vi "SwitchesMirrors.vi"(0 "Function":T5, 5 "Relay VISA Session":refnum<visa-resource-name>="COM1", 7 "Set Switch":T1, 9 "Delays (ms)":cluster{"Laser":u32, "Video":u32}={"Laser"=500, "Video"=1500}, 11 "Error In":errorcluster, 13 "Refnums":T4, 14 "Notifiers":T3) -> (8 "Get Switch":T1, 15 "Error Out":errorcluster)   [LabVIEW 2014]
uses:
  SwitchesMirrors Functions.ctl
  SwitchesMirrors Refnum.ctl
  support/Instrument Status.ctl
  SwitchesMirrors Notifiers.ctl
  SwitchesMirrors Status.ctl
  support/Instrument Status State.ctl
panel:
  out "Instrument Status":T2
  # "LICENSED MATERIALS – PROPERTY OF IBM\nCopyright IBM Corp. 2016,\nALL RIGHTS RESERVED"
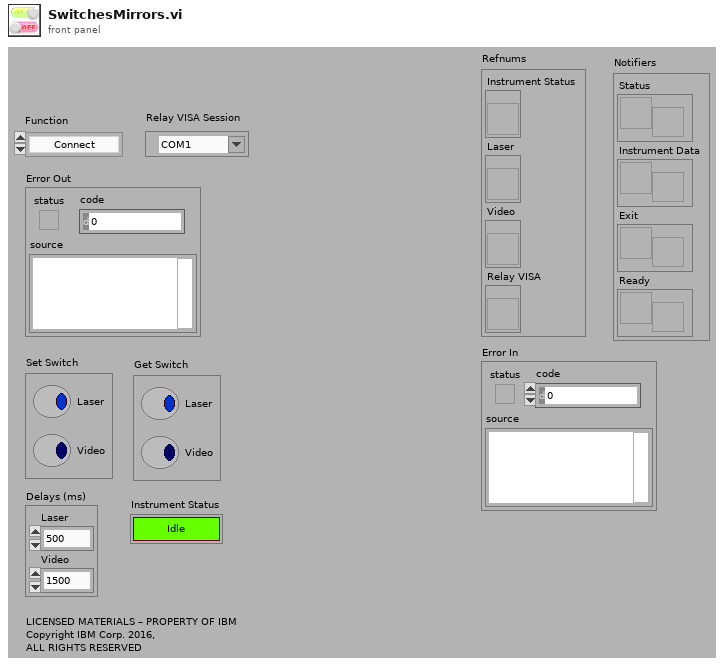
[diagram p1: front panel]
types:
  T1 = typedef "SwitchesMirrors Status.ctl" = cluster{"Laser":bool, "Video":bool}
  T2 = typedef "Instrument Status.ctl" = bool
  T3 = typedef "SwitchesMirrors Notifiers.ctl" = cluster{"Status":refnum<notifier>, "Instrument Data":refnum<notifier>, "Exit":refnum<notifier>, "Ready":refnum<notifier>}
  T4 = typedef "SwitchesMirrors Refnum.ctl" = cluster{"Instrument Status":refnum<vi>, "Laser":refnum<vi>, "Video":refnum<vi>, "Relay VISA":refnum<vi>}
  T5 = typedef "SwitchesMirrors Functions.ctl" = enum16{"Connect", "Get Configuration", "Set Configuration", "Update Refnums", "Disconnect"}
  T6 = enum16{"Connect", "Generic I/O", "Initialize", "Get Configuration", "Switch Relay", "Info", "Disconnect"}
  T7 = typedef "Instrument Status State.ctl" = enum16{"Unknown", "Idle", "Standby", "Configuring", "Measuring", "Moving", "Disconnected"}
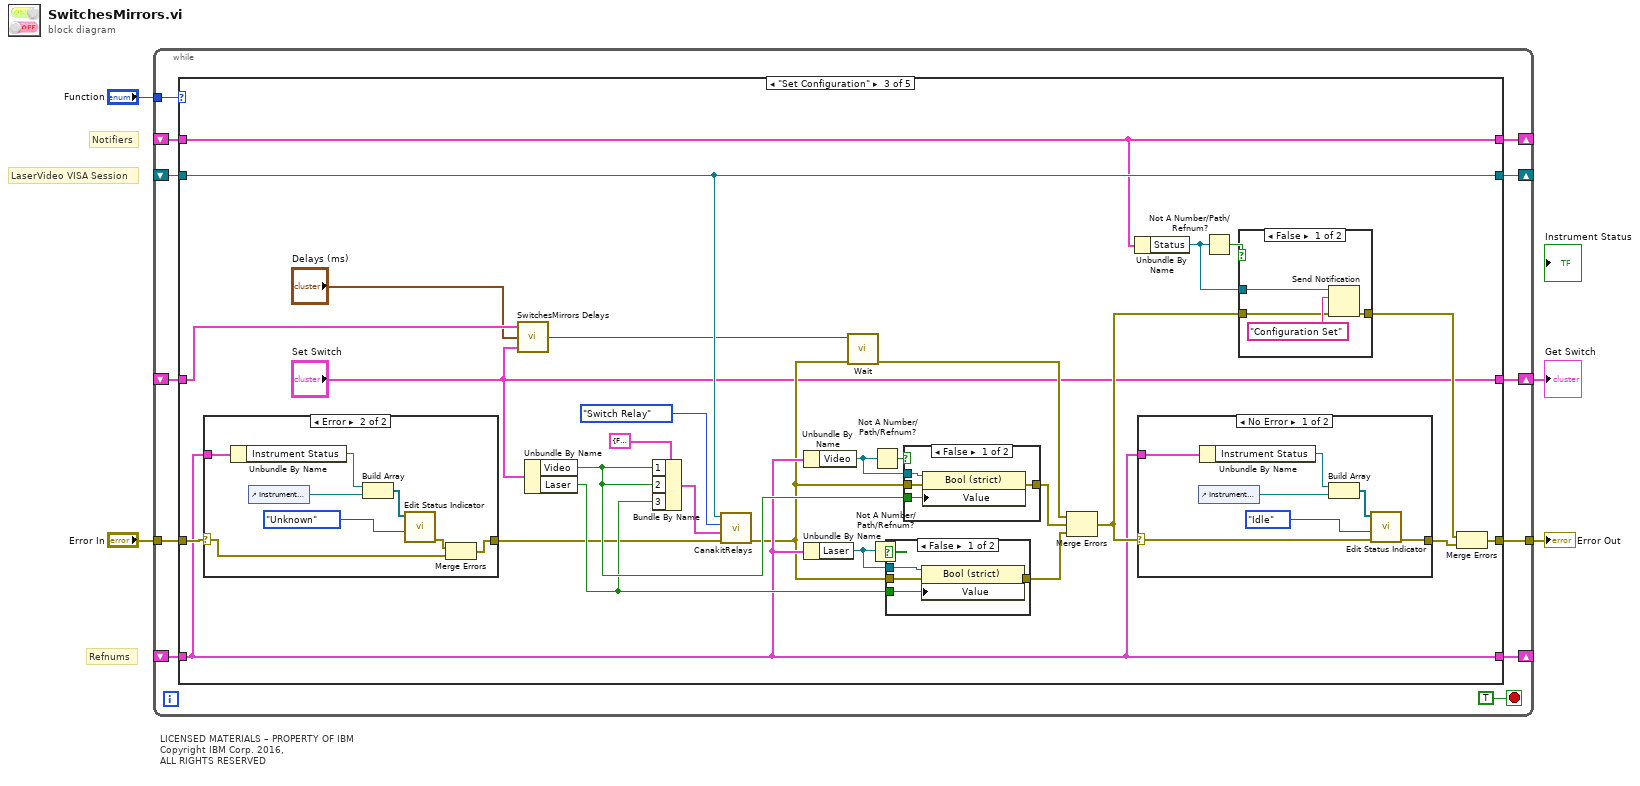
[diagram p0: block diagram]
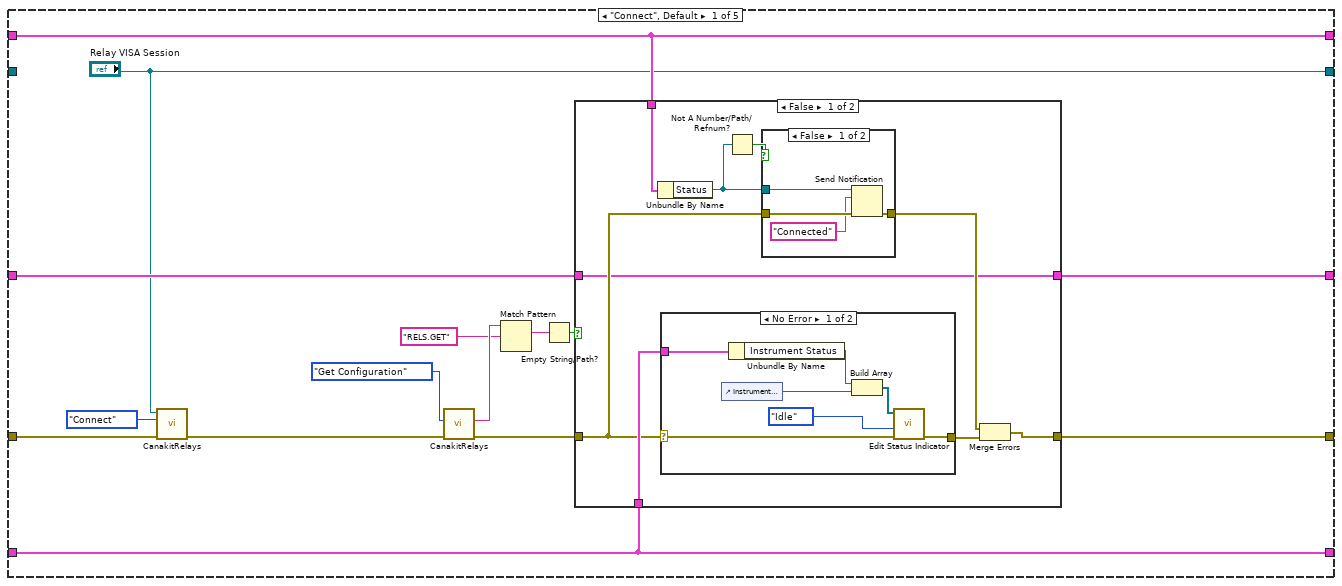
[diagram p2: hidden frame]
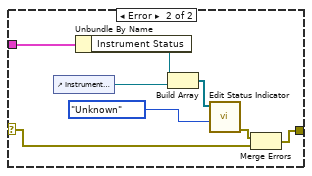
[diagram p3: hidden frame]
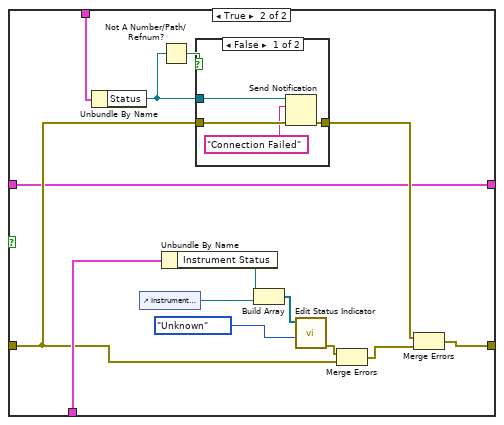
[diagram p5: hidden frame]
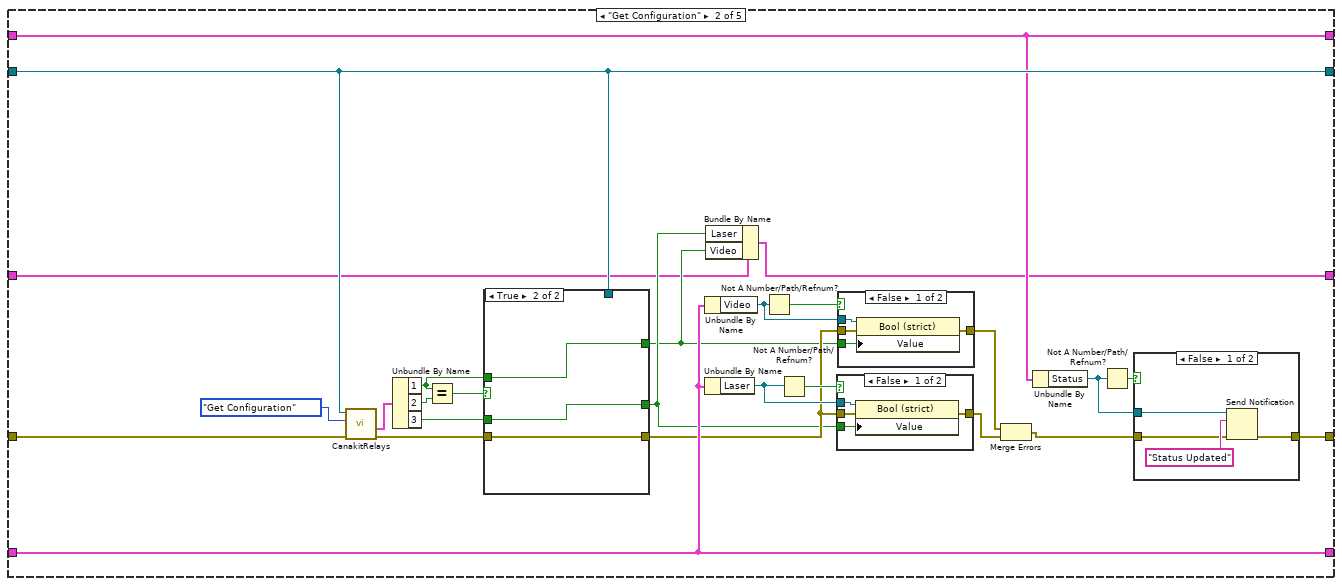
[diagram p7: hidden frame]
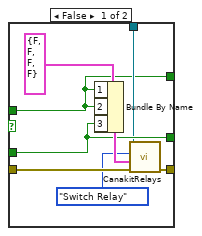
[diagram p11: hidden frame]
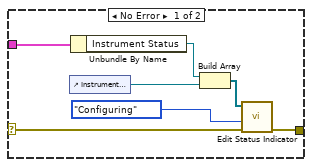
[diagram p12: hidden frame]
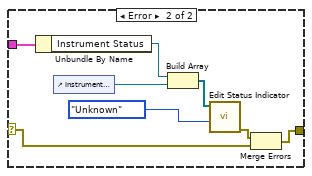
[diagram p13: hidden frame]
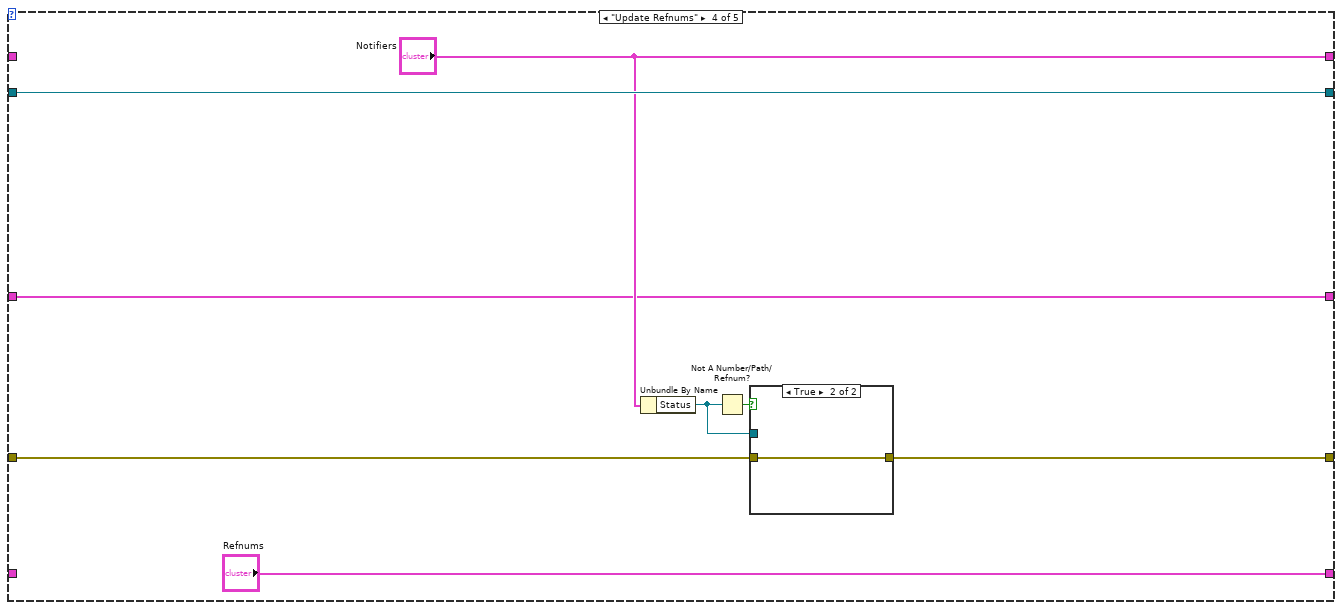
[diagram p17: hidden frame]
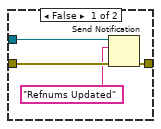
[diagram p18: hidden frame]
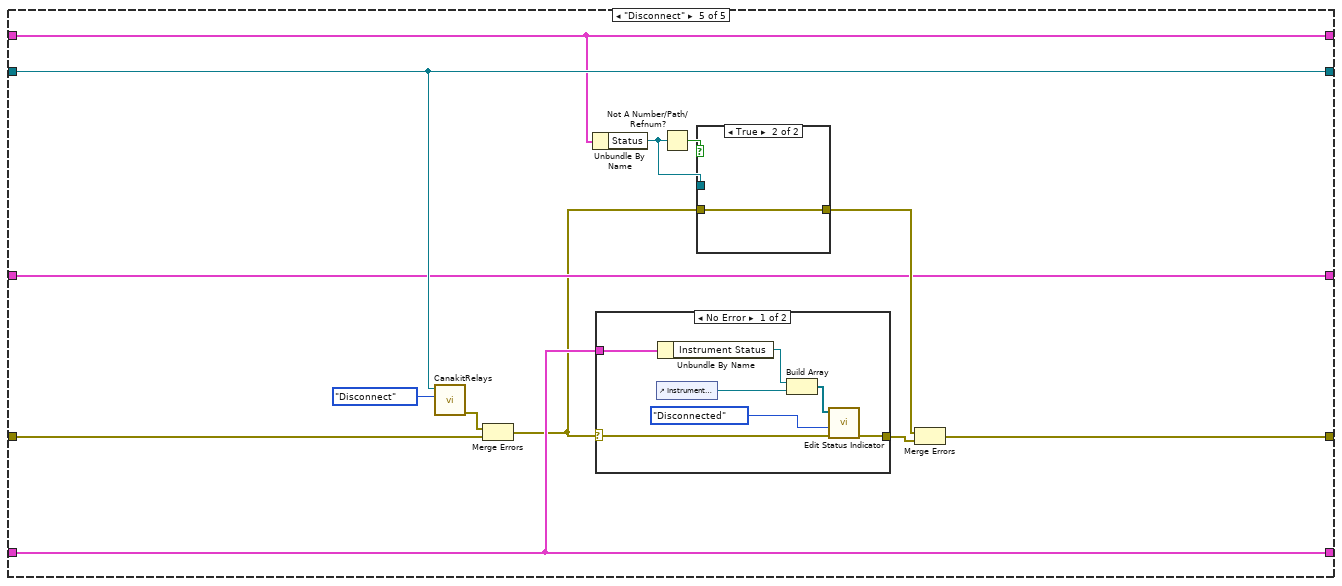
[diagram p19: hidden frame]
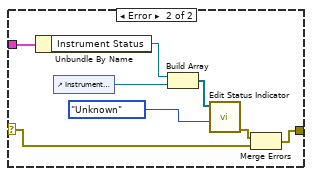
[diagram p20: hidden frame]
diagram:
  # "LICENSED MATERIALS – PROPERTY OF IBM\nCopyright IBM Corp. 2016,\nALL RIGHTS RESERVED"
  # "Notifiers"
  # "LaserVideo VISA Session"
  # "Refnums"
  n1 = while {
    tunnel: [w16] -> w4
    tunnel: "Error In" -> [w15]
    shift-right: [w12] -> _
    shift-left: _ -> [w11]
    tunnel: "Function" -> [w13]
    shift-right: [w10] -> _
    shift-left: _ -> [w9]
    shift-right: [w7] -> _
    shift-left: _ -> [w8]
    shift-right: [w6] -> w1
    shift-left: _ -> [w5]
    stop <- TRUE stop-if-true
    n2 = case shown="\"Set Configuration\"" w13 {
      tunnel: [w28 w84 w142 w206 w221] -> w16
      tunnel: w15 -> [w31 w100 w141 w207 w218]
      tunnel: ["Relay VISA Session" w99 w157 w212 w230] -> w12
      tunnel: w11 -> [_ w99 w157 w212 w230]
      tunnel: [w30 w96 w140 "Refnums" w222] -> w10
      tunnel: w9 -> [w30 w96 w140 _ w222]
      tunnel: w8 -> [w29 w86 w144 _ w224]
      tunnel: [w29 w86 w144 "Notifiers" w224] -> w7
      tunnel: [w23 w82 "Set Switch" w205 w220] -> w6
      tunnel: w5 -> [w25 w81 w135 w205 w220]
      frame "Connect", Default {
        n3 = call "CanakitRelays.vi"("Error In"=w31, "Function"=T6."Connect", "VISA resource name"="Relay VISA Session") -> ("Error Out"=w17:errorcluster)  [unwired: 2 in, 6 out]
        n4 = call "CanakitRelays.vi"("Error In"=w17, "Function"=T6."Get Configuration") -> ("Error Out"=w26:errorcluster, "Read String"=w21:string)  [unwired: 3 in, 5 out]
        n5 = Match Pattern(string=w21, regular expression="RELS.GET") -> (match substring=w19:string)  [unwired: 1 in, 3 out]
        n6 = Empty String/Path?(string/path=w19) -> (empty?=w24:bool)
        n7 = case shown="False" w24 {
          tunnel: w30 -> [w38 w72]
          tunnel: w29 -> [w37 w71]
          tunnel: [w36 w70] -> w28
          tunnel: w26 -> [w33 w67]
          tunnel: w25 -> [w32 w66]
          tunnel: [w32 w66] -> w23
          frame False {
            n8 = Unbundle By Name(w37) -> ("Status"=w39:refnum<notifier>)
            n9 = case shown="No Error" w33 {
              selector: w33 -> [w46 w50]
              tunnel: [w45 w49] -> w34
              tunnel: w38 -> [w41 w51]
              frame No Error {
                n10 = control-ref of="Instrument Status"() -> (w44:refnum<vi>)
                n11 = Unbundle By Name(w41) -> ("Instrument Status"=w42:refnum<vi>)
                n12 = Build Array(w42, w44) -> (w43:refnum<vi>[])
                n13 = call "Edit Status Indicator.vi"("error in (no error)"=w46, "State"=Instrument_Status_State."Idle", "Instrument Status Refnum"=w43) -> ("error out"=w45:errorcluster)  [unwired: 1 in, 7 out]
              }
              frame Error {
                n14 = control-ref of="Instrument Status"() -> (w54:refnum<vi>)
                n15 = Unbundle By Name(w51) -> ("Instrument Status"=w52:refnum<vi>)
                n16 = Build Array(w52, w54) -> (w53:refnum<vi>[])
                n17 = call "Edit Status Indicator.vi"("State"=Instrument_Status_State."Unknown", "Instrument Status Refnum"=w53) -> ("error out"=w48:errorcluster)  [unwired: 2 in, 7 out]
                n18 = Merge Errors(w48, w50) -> (w49:errorcluster)
              }
            }
            n19 = Not A Number/Path/Refnum?(number/path/refnum=w39) -> (NaN/Path/Refnum?=w40:bool)
            n20 = case shown="False" w40 {
              tunnel: w33 -> [w59 w60]
              tunnel: [w58 w60] -> w35
              tunnel: w39 -> [w57 _]
              frame False {
                n21 = Send Notification(notification="Connected", notifier=w57, error in (no error)=w59) -> (error out=w58:errorcluster)  [unwired: 1 out]
              }
              frame True {
              }
            }
            n22 = Merge Errors(w35, w34) -> (w36:errorcluster)
          }
          frame True {
            n23 = Unbundle By Name(w71) -> ("Status"=w73:refnum<notifier>)
            n24 = control-ref of="Instrument Status"() -> (w64:refnum<vi>)
            n25 = Not A Number/Path/Refnum?(number/path/refnum=w73) -> (NaN/Path/Refnum?=w74:bool)
            n26 = Unbundle By Name(w72) -> ("Instrument Status"=w62:refnum<vi>)
            n27 = case shown="False" w74 {
              tunnel: w67 -> [w78 w79]
              tunnel: [w77 w79] -> w69
              tunnel: w73 -> [w76 _]
              frame False {
                n28 = Send Notification(notification="Connection Failed", notifier=w76, error in (no error)=w78) -> (error out=w77:errorcluster)  [unwired: 1 out]
              }
              frame True {
              }
            }
            n29 = Build Array(w62, w64) -> (w63:refnum<vi>[])
            n30 = call "Edit Status Indicator.vi"("State"=Instrument_Status_State."Unknown", "Instrument Status Refnum"=w63) -> ("error out"=w61:errorcluster)  [unwired: 2 in, 7 out]
            n31 = Merge Errors(w61, w67) -> (w68:errorcluster)
            n32 = Merge Errors(w69, w68) -> (w70:errorcluster)
          }
        }
      }
      frame "Get Configuration" {
        n33 = call "CanakitRelays.vi"("Error In"=w100, "Function"=T6."Get Configuration", "VISA resource name"=w99) -> ("Error Out"=w102:errorcluster, "Get Relays"=w104:cluster{"1":bool, "2":bool, "3":bool, "4":bool})  [unwired: 2 in, 5 out]
        n34 = Unbundle By Name(w104) -> ("1"=w80:bool, "2"=w105:bool, "3"=w101:bool)
        n35 = Equal?(x=w80, y=w105) -> (x = y?=w103:bool)
        n36 = case shown="True" w103 {
          tunnel: w102 -> [w128 w131]
          tunnel: [w127 w131] -> w91
          tunnel: w101 -> [w124 w130]
          tunnel: [w121 w129] -> w89
          tunnel: [w124 w130] -> w90
          tunnel: w99 -> [w123 _]
          tunnel: w80 -> [w121 w129]
          frame False {
            n37 = Bundle By Name(cluster=cluster{"1":bool, "2":bool, "3":bool, "4":bool} {"1"=FALSE, "2"=FALSE, "3"=FALSE, "4"=FALSE} ("Relays"), "1"=w121, "2"=w121, "3"=w124) -> (w126:cluster{"1":bool, "2":bool, "3":bool, "4":bool})
            n38 = call "CanakitRelays.vi"("Error In"=w128, "Set Relays"=w126, "Function"=T6."Switch Relay", "VISA resource name"=w123) -> ("Error Out"=w127:errorcluster)  [unwired: 1 in, 6 out]
          }
          frame True {
          }
        }
        n39 = Unbundle By Name(w96) -> ("Video"=w97:refnum<vi>)
        n40 = Unbundle By Name(w96) -> ("Laser"=w94:refnum<vi>)
        n41 = Bundle By Name(cluster=w81, "Laser"=w90, "Video"=w89) -> (w82:T1)
        n42 = Not A Number/Path/Refnum?(number/path/refnum=w97) -> (NaN/Path/Refnum?=w98:bool)
        n43 = Not A Number/Path/Refnum?(number/path/refnum=w94) -> (NaN/Path/Refnum?=w95:bool)
        n44 = case shown="False" w95 {
          tunnel: w90 -> [w114 _]
          tunnel: w94 -> [w113 _]
          tunnel: [w112 w115] -> w93
          tunnel: w91 -> [w111 w115]
          frame False {
            n45 = property class="Bool (strict)"(reference=w113, error in=w111, "Value"=w114) -> (error out=w112:errorcluster)  [unwired: 1 out]
          }
          frame True {
          }
        }
        n46 = case shown="False" w98 {
          tunnel: w89 -> [w119 _]
          tunnel: w97 -> [w118 _]
          tunnel: [w117 w120] -> w92
          tunnel: w91 -> [w116 w120]
          frame False {
            n47 = property class="Bool (strict)"(reference=w118, error in=w116, "Value"=w119) -> (error out=w117:errorcluster)  [unwired: 1 out]
          }
          frame True {
          }
        }
        n48 = Merge Errors(w92, w93) -> (w85:errorcluster)
        n49 = Unbundle By Name(w86) -> ("Status"=w87:refnum<notifier>)
        n50 = Not A Number/Path/Refnum?(number/path/refnum=w87) -> (NaN/Path/Refnum?=w88:bool)
        n51 = case shown="False" w88 {
          tunnel: [w109 w110] -> w84
          tunnel: w87 -> [w108 _]
          tunnel: w85 -> [w106 w110]
          frame False {
            n52 = Send Notification(notification="Status Updated", notifier=w108, error in (no error)=w106) -> (error out=w109:errorcluster)  [unwired: 1 out]
          }
          frame True {
          }
        }
      }
      frame "Set Configuration" {
        n53 = case shown="Error" w141 {
          selector: w141 -> [w165 w171]
          tunnel: [w164 w170] -> w138
          tunnel: w140 -> [w160 w167]
          frame No Error {
            n54 = control-ref of="Instrument Status"() -> (w163:refnum<vi>)
            n55 = Unbundle By Name(w160) -> ("Instrument Status"=w161:refnum<vi>)
            n56 = Build Array(w161, w163) -> (w162:refnum<vi>[])
            n57 = call "Edit Status Indicator.vi"("error in (no error)"=w165, "State"=Instrument_Status_State."Configuring", "Instrument Status Refnum"=w162) -> ("error out"=w164:errorcluster)  [unwired: 1 in, 7 out]
          }
          frame Error {
            n58 = Unbundle By Name(w167) -> ("Instrument Status"=w168:refnum<vi>)
            n59 = control-ref of="Instrument Status"() -> (w173:refnum<vi>)
            n60 = Build Array(w168, w173) -> (w172:refnum<vi>[])
            n61 = call "Edit Status Indicator.vi"("State"=Instrument_Status_State."Unknown", "Instrument Status Refnum"=w172) -> ("error out"=w169:errorcluster)  [unwired: 2 in, 7 out]
            n62 = Merge Errors(w169, w171) -> (w170:errorcluster)
          }
        }
        n63 = call "SwitchesMirrors Delays.vi"("Set Switch"="Set Switch", "Delays (ms)"="Delays (ms)", "Status"=w135) -> ("Delay"=w132:u32)  [unwired: 1 in]
        n64 = Unbundle By Name("Set Switch") -> ("Video"=w150:bool, "Laser"=w149:bool)
        n65 = Bundle By Name(cluster=cluster{"1":bool, "2":bool, "3":bool, "4":bool} {"1"=FALSE, "2"=FALSE, "3"=FALSE, "4"=FALSE} ("Relays"), "1"=w150, "2"=w150, "3"=w149) -> (w158:cluster{"1":bool, "2":bool, "3":bool, "4":bool})
        n66 = call "CanakitRelays.vi"("Error In"=w138, "Set Relays"=w158, "Function"=T6."Switch Relay", "VISA resource name"=w157) -> ("Error Out"=w136:errorcluster)  [unwired: 1 in, 6 out]
        n67 = Unbundle By Name(w140) -> ("Video"=w155:refnum<vi>)
        n68 = Unbundle By Name(w140) -> ("Laser"=w153:refnum<vi>)
        n69 = call "Wait.vi"("error in (no error)"=w136, "milliseconds to wait"=w132) -> ("error out"=w137:errorcluster)  [unwired: 9 in]
        n70 = Not A Number/Path/Refnum?(number/path/refnum=w153) -> (NaN/Path/Refnum?=w154:bool)
        n71 = Not A Number/Path/Refnum?(number/path/refnum=w155) -> (NaN/Path/Refnum?=w156:bool)
        n72 = case shown="False" w154 {
          tunnel: w149 -> [w198 _]
          tunnel: w153 -> [w197 _]
          tunnel: [w196 w199] -> w152
          tunnel: w136 -> [w195 w199]
          frame False {
            n73 = property class="Bool (strict)"(reference=w197, error in=w195, "Value"=w198) -> (error out=w196:errorcluster)  [unwired: 1 out]
          }
          frame True {
          }
        }
        n74 = case shown="False" w156 {
          tunnel: w150 -> [w203 _]
          tunnel: w155 -> [w202 _]
          tunnel: [w201 w204] -> w151
          tunnel: w136 -> [w200 w204]
          frame False {
            n75 = property class="Bool (strict)"(reference=w202, error in=w200, "Value"=w203) -> (error out=w201:errorcluster)  [unwired: 1 out]
          }
          frame True {
          }
        }
        n76 = Merge Errors(w137, w151, w152) -> (w143:errorcluster)
        n77 = Unbundle By Name(w144) -> ("Status"=w145:refnum<notifier>)
        n78 = case shown="No Error" w143 {
          selector: w143 -> [w180 w186]
          tunnel: [w179 w185] -> w146
          tunnel: w140 -> [w175 w183]
          frame No Error {
            n79 = control-ref of="Instrument Status"() -> (w178:refnum<vi>)
            n80 = Unbundle By Name(w175) -> ("Instrument Status"=w176:refnum<vi>)
            n81 = Build Array(w176, w178) -> (w177:refnum<vi>[])
            n82 = call "Edit Status Indicator.vi"("error in (no error)"=w180, "State"=Instrument_Status_State."Idle", "Instrument Status Refnum"=w177) -> ("error out"=w179:errorcluster)  [unwired: 1 in, 7 out]
          }
          frame Error {
            n83 = Unbundle By Name(w183) -> ("Instrument Status"=w182:refnum<vi>)
            n84 = control-ref of="Instrument Status"() -> (w188:refnum<vi>)
            n85 = Build Array(w182, w188) -> (w187:refnum<vi>[])
            n86 = call "Edit Status Indicator.vi"("State"=Instrument_Status_State."Unknown", "Instrument Status Refnum"=w187) -> ("error out"=w184:errorcluster)  [unwired: 2 in, 7 out]
            n87 = Merge Errors(w184, w186) -> (w185:errorcluster)
          }
        }
        n88 = Not A Number/Path/Refnum?(number/path/refnum=w145) -> (NaN/Path/Refnum?=w148:bool)
        n89 = case shown="False" w148 {
          tunnel: [w193 w194] -> w147
          tunnel: w145 -> [w191 _]
          tunnel: w143 -> [w190 w194]
          frame False {
            n90 = Send Notification(notification="Configuration Set", notifier=w191, error in (no error)=w190) -> (error out=w193:errorcluster)  [unwired: 1 out]
          }
          frame True {
          }
        }
        n91 = Merge Errors(w147, w146) -> (w142:errorcluster)
      }
      frame "Update Refnums" {
        n92 = Unbundle By Name("Notifiers") -> ("Status"=w210:refnum<notifier>)
        n93 = Not A Number/Path/Refnum?(number/path/refnum=w210) -> (NaN/Path/Refnum?=w209:bool)
        n94 = case shown="True" w209 {
          tunnel: w207 -> [w216 w217]
          tunnel: [w215 w217] -> w206
          tunnel: w210 -> [w214 _]
          frame False {
            n95 = Send Notification(notification="Refnums Updated", notifier=w214, error in (no error)=w216) -> (error out=w215:errorcluster)  [unwired: 1 out]
          }
          frame True {
          }
        }
      }
      frame "Disconnect" {
        n96 = call "CanakitRelays.vi"("Function"=T6."Disconnect", "VISA resource name"=w230) -> ("Error Out"=w223:errorcluster)  [unwired: 3 in, 6 out]
        n97 = Merge Errors(w223, w218) -> (w219:errorcluster)
        n98 = Unbundle By Name(w224) -> ("Status"=w225:refnum<notifier>)
        n99 = case shown="No Error" w219 {
          selector: w219 -> [w236 w242]
          tunnel: [w235 w241] -> w226
          tunnel: w222 -> [w231 w239]
          frame No Error {
            n100 = control-ref of="Instrument Status"() -> (w234:refnum<vi>)
            n101 = Unbundle By Name(w231) -> ("Instrument Status"=w232:refnum<vi>)
            n102 = Build Array(w232, w234) -> (w233:refnum<vi>[])
            n103 = call "Edit Status Indicator.vi"("error in (no error)"=w236, "State"=Instrument_Status_State."Disconnected", "Instrument Status Refnum"=w233) -> ("error out"=w235:errorcluster)  [unwired: 1 in, 7 out]
          }
          frame Error {
            n104 = Unbundle By Name(w239) -> ("Instrument Status"=w238:refnum<vi>)
            n105 = control-ref of="Instrument Status"() -> (w244:refnum<vi>)
            n106 = Build Array(w238, w244) -> (w243:refnum<vi>[])
            n107 = call "Edit Status Indicator.vi"("State"=Instrument_Status_State."Unknown", "Instrument Status Refnum"=w243) -> ("error out"=w240:errorcluster)  [unwired: 2 in, 7 out]
            n108 = Merge Errors(w240, w242) -> (w241:errorcluster)
          }
        }
        n109 = Not A Number/Path/Refnum?(number/path/refnum=w225) -> (NaN/Path/Refnum?=w228:bool)
        n110 = case shown="True" w228 {
          tunnel: [w249 w250] -> w227
          tunnel: w225 -> [w247 _]
          tunnel: w219 -> [w246 w250]
          frame False {
            n111 = Send Notification(notification="Disconnected", notifier=w247, error in (no error)=w246) -> (error out=w249:errorcluster)  [unwired: 1 out]
          }
          frame True {
          }
        }
        n112 = Merge Errors(w227, w226) -> (w221:errorcluster)
      }
    }
  }
  "Error Out" <- w4
  "Get Switch" <- w1
